vi "String to bit (SubVI).vi"(11 "String in":string) -> (1 "Pointy finger":dbl, 2 "Middle finger":dbl, 3 "Ringfinger":dbl, 4 "Thumb":dbl, 5 "Lillfinger":dbl, 6 "Command LSD":dbl, 7 "Command MSD":dbl)   [LabVIEW 2016]
uses:
  <vilib>/express/express arith-compare/Formula/XNode/ExpressFormulaBlockNode.xnode
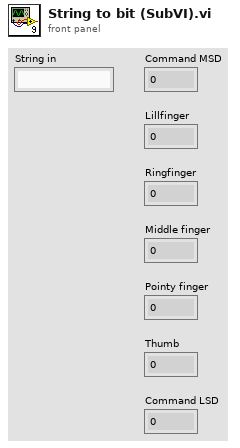
[diagram p1: front panel]
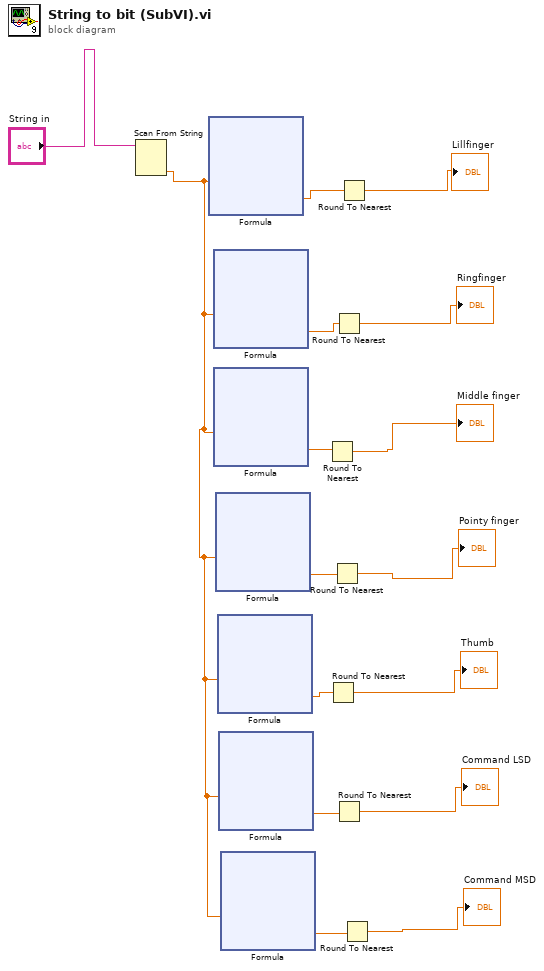
[diagram p0: block diagram]
diagram:
  n1 = Scan From String(input string="String in") -> (output 1=w15:dbl)  [unwired: 4 in, 3 out]
  n2 = xnode "Formula"("X1"=w15) -> ("Result"=w14:dbl)  [unwired: 1 in, 1 out]
  n3 = xnode "Formula"("X1"=w15) -> ("Result"=w6:dbl)  [unwired: 1 in, 1 out]
  n4 = xnode "Formula"("X1"=w15) -> ("Result"=w5:dbl)  [unwired: 1 in, 1 out]
  n5 = xnode "Formula"("X1"=w15) -> ("Result"=w4:dbl)  [unwired: 1 in, 1 out]
  n6 = xnode "Formula"("X1"=w15) -> ("Result"=w3:dbl)  [unwired: 1 in, 1 out]
  n7 = xnode "Formula"("X1"=w15) -> ("Result"=w2:dbl)  [unwired: 1 in, 1 out]
  n8 = xnode "Formula"("X1"=w15) -> ("Result"=w1:dbl)  [unwired: 1 in, 1 out]
  n9 = Round To Nearest(number=w5) -> (nearest integer value=→"Middle finger":dbl)
  n10 = Round To Nearest(number=w3) -> (nearest integer value=→"Thumb":dbl)
  n11 = Round To Nearest(number=w4) -> (nearest integer value=→"Pointy finger":dbl)
  n12 = Round To Nearest(number=w6) -> (nearest integer value=→"Ringfinger":dbl)
  n13 = Round To Nearest(number=w2) -> (nearest integer value=→"Command LSD":dbl)
  n14 = Round To Nearest(number=w14) -> (nearest integer value=→"Lillfinger":dbl)
  n15 = Round To Nearest(number=w1) -> (nearest integer value=→"Command MSD":dbl)
